vi "InitializationRoutine.vi"(8 "error in (no error)":errorcluster, 9 "Start microPython?":bool=TRUE, 10 "py file":path, 11 "Refnum in":refnum<k35>) -> (0 "error out":errorcluster, 1 "source":string="\n\n", 3 "Refnum out":refnum<k35>)   [LabVIEW 2019]
uses:
  <vilib>/Utility/error.llb/DialogType.ctl
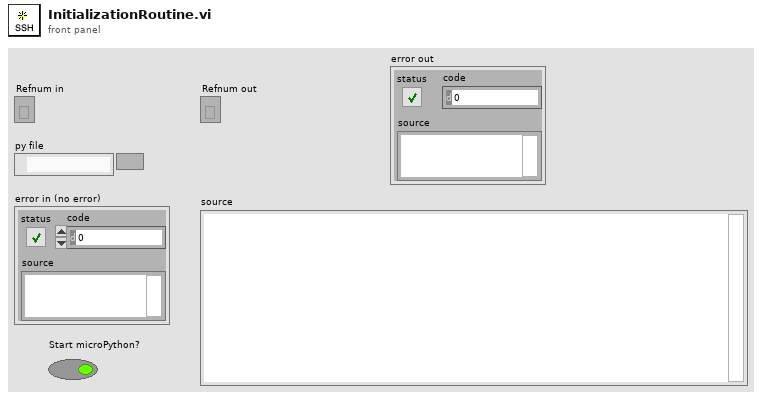
[diagram p1: front panel]
types:
  T1 = typedef "DialogType.ctl" = u16
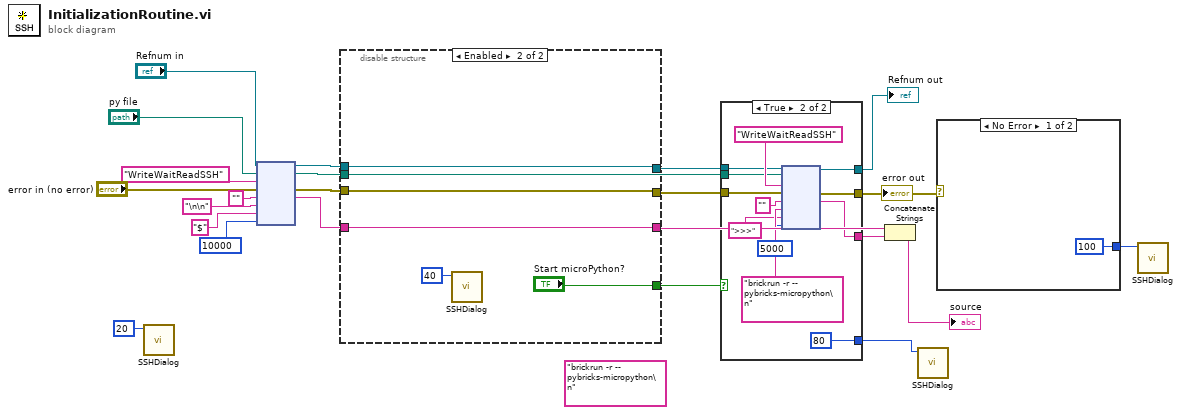
[diagram p0: block diagram]
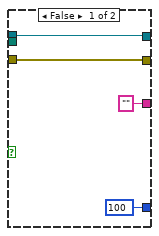
[diagram p2: hidden frame]
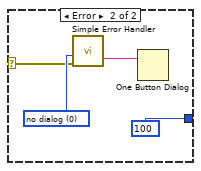
[diagram p3: hidden frame]
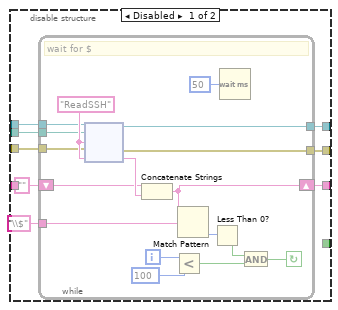
[diagram p4: hidden frame]
diagram:
  (unwired) "brickrun -r --  pybricks-micropython\n" ("function name")
  n1 = call <userlib>:"SSHDialog.vi"("Slide"=u8 20) -> ()  [unwired: 11 in]
  n2 = node("Refnum in", "py file", "WriteWaitReadSSH" ("function name"), "error in (no error)", "" ("function name"), "\n\n" ("function name"), "$" ("EOL"), u32 10000 ("milliseconds to wait")) -> (w17:refnum<k35>, w15:errorcluster, w8:string)  [unwired: 3 in, 2 out]
  n3 = disable-structure shown="Enabled" {
    disable-tunnel: w17 -> [w30 w52]
    disable-tunnel: [w29 w52] -> w16
    disable-tunnel: w15 -> [w28 w51]
    disable-tunnel: [w27 w51] -> w14
    disable-tunnel: "py file" -> [w26 _]
    disable-tunnel: [w25 w50] -> w6
    disable-tunnel: w8 -> [_ w50]
    disable-tunnel: [_ "Start microPython?"] -> w7
    frame Disabled {
      n4 = while {
        tunnel: w30 -> [w46]
        tunnel: [w45] -> w29
        tunnel: w28 -> [w44]
        tunnel: [w43] -> w27
        tunnel: w26 -> [w42]
        shift-right: [w39] -> w25
        shift-left: "" -> [w40]
        tunnel: "\\$" ("regular expression") -> [w31]
        i -> [w36]
        stop <- w32 continue-if-true
        w47 = "ReadSSH" ("function name")
        # "wait for $"
        n5 = node(w46, w42, w47, w44, w47) -> (w45:refnum<k35>, w43:errorcluster, w41:string)  [unwired: 2 out]
        n6 = Concatenate Strings(w40, w41) -> (w39:string)
        n7 = Less?(x=w36, y=100) -> (x < y?=w33:bool)
        n8 = Match Pattern(string=w39, regular expression=w31) -> (offset past match=w38:i32)  [unwired: 1 in, 3 out]
        n9 = Less Than 0?(x=w38) -> (x < 0?=w34:bool)
        n10 = Wait (ms)(milliseconds to wait=u32 50) -> ()  [unwired: 1 out]
        n11 = And(x=w34, y=w33) -> (x .and. y?=w32:bool)
      }
    }
    frame Enabled {
      n12 = call <userlib>:"SSHDialog.vi"("Slide"=u8 40) -> ()  [unwired: 11 in]
    }
  }
  n13 = case shown="True" w7 {
    tunnel: w16 -> [w56 w65]
    tunnel: w14 -> [w55 w64]
    tunnel: [w56 w63] -> w13
    tunnel: "py file" -> [_ w62]
    tunnel: [w55 w61] -> w11
    tunnel: ["" ("function name") w58] -> w5
    tunnel: [u8 100 ("Slide") u8 80 ("Slide")] -> w3
    frame False {
    }
    frame True {
      n14 = node(w65, w62, "WriteWaitReadSSH" ("function name"), w64, "" ("function name"), "brickrun -r --  pybricks-micropython\n" ("function name"), ">>>" ("EOL"), u32 5000 ("milliseconds to wait")) -> (w63:refnum<k35>, w61:errorcluster, w58:string)  [unwired: 3 in, 2 out]
    }
  }
  "Refnum out" <- w13
  "error out" <- w11
  n15 = Concatenate Strings(w6, w5) -> (→"source":string)
  n16 = call <userlib>:"SSHDialog.vi"("Slide"=w3) -> ()  [unwired: 11 in]
  n17 = case shown="No Error" w11 {
    selector: w11 -> [_ w72]
    tunnel: [u8 100 ("Slide") u8 100 ("Slide")] -> w2
    frame No Error {
    }
    frame Error {
      w73 = T1 0 items=["no dialog", "OK message", "continue or stop message", "OK message + warnings", "continue/stop + warnings"] ("type of dialog (OK msg:1)")
      n18 = call <vilib>:"Simple Error Handler.vi"("type of dialog (OK msg:1)"=w73, "error in (no error)"=w72) -> ("message"=w71:string)  [unwired: 3 in, 4 out]
      n19 = One Button Dialog(message=w71) -> ()  [unwired: 1 in, 1 out]
    }
  }
  n20 = call <userlib>:"SSHDialog.vi"("Slide"=w2) -> ()  [unwired: 11 in]
